vi "CMH_Data_seperation.vi"(11 "Humidity readout":string) -> (0 "??":string, 1 "AT":dbl, 2 "AT[C]":string, 3 "read buffer":string, 4 "RH":dbl, 5 "DP":dbl, 6 "RH[%]":string, 7 "DP[C]":string)   [LabVIEW 2024]
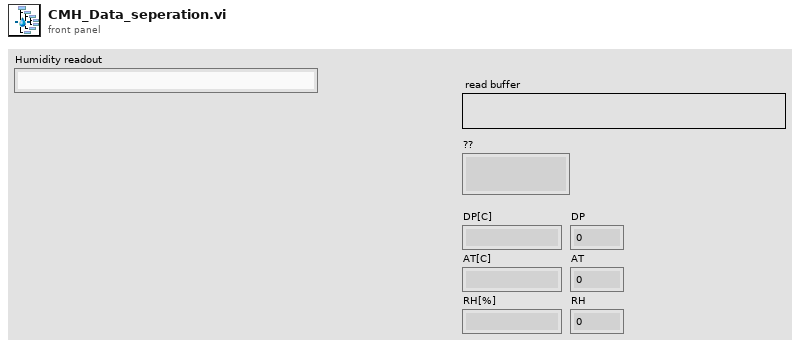
[diagram p1: front panel]
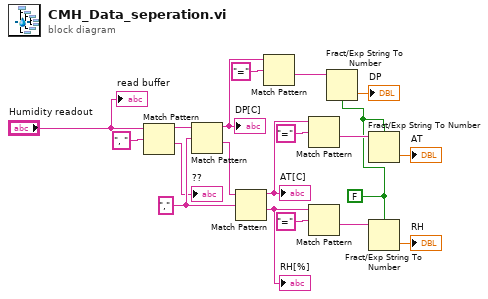
[diagram p0: block diagram]
diagram:
  w1 = FALSE ("use system decimal point (T)")
  w18 = "," ("search string/char (-)")
  n1 = Match Pattern(string="Humidity readout", regular expression=", ") -> (before substring=w15:string, after substring=→"??":string)  [unwired: 1 in, 2 out]
  n2 = Match Pattern(string=w15, regular expression=w18) -> (before substring=w14:string, after substring=w19:string)  [unwired: 1 in, 2 out]
  "DP[C]" <- w14
  n3 = Match Pattern(string=w19, regular expression=w18) -> (before substring=w10:string, after substring=w8:string)  [unwired: 1 in, 2 out]
  "AT[C]" <- w10
  "RH[%]" <- w8
  n4 = Match Pattern(string=w14, regular expression="=") -> (after substring=w7:string)  [unwired: 1 in, 3 out]
  n5 = Match Pattern(string=w10, regular expression="=") -> (after substring=w5:string)  [unwired: 1 in, 3 out]
  n6 = Match Pattern(string=w8, regular expression="=") -> (after substring=w3:string)  [unwired: 1 in, 3 out]
  n7 = Fract/Exp String To Number(use system decimal point (T)=w1, string=w7) -> (number=→"DP":dbl)  [unwired: 2 in, 1 out]
  n8 = Fract/Exp String To Number(use system decimal point (T)=w1, string=w5) -> (number=→"AT":dbl)  [unwired: 2 in, 1 out]
  n9 = Fract/Exp String To Number(use system decimal point (T)=w1, string=w3) -> (number=→"RH":dbl)  [unwired: 2 in, 1 out]
  "read buffer" <- "Humidity readout"
